vi "RefnumGlobal.vi"() -> ()   [LabVIEW 2009, in "ListImp_RefSpy.lvclass"]
uses:
  ListImp_RefSpy.lvclass
panel:
  in  "MethodsCalled":string[](array[string])
  in  "Refnum":refnum<queue>
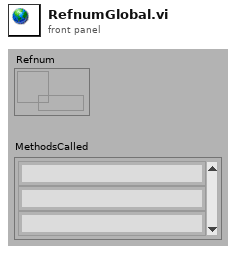
[diagram p1: front panel]
diagram:
